vi "Exit.vi"(8 "error in (no error)":errorcluster, 11 "Old State":refnum<class "New_Transaction.lvclass">) -> (0 "error out":errorcluster, 3 "New State":refnum<class "New_Transaction.lvclass">)   [LabVIEW 2025, in "User_Console-ATM.lvlib" / "New_Transaction.lvclass"]
doc: "This is an abstract method. Override this method to define the behavior when you leave the state."
uses:
  New_Transaction.lvclass
  New_Transaction.lvclass/New_Transaction.ctl
  User_Console_States/User_Console_States.lvclass
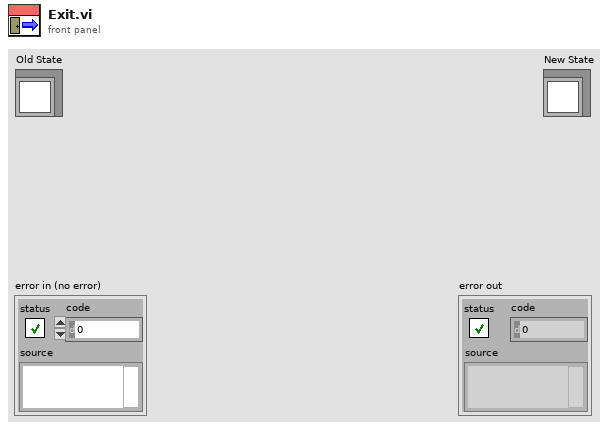
[diagram p1: front panel]
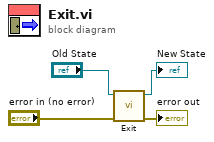
[diagram p0: block diagram]
diagram:
  n1 = call-parent "Exit.vi"("error in (no error)"="error in (no error)", "Old State"="Old State") -> ("error out"=→"error out":errorcluster, "New State"=→"New State":refnum<class "New_Transaction.lvclass">)  [unwired: 8 in]
